vi "kill VSC debug port.vi"(8 "error in (no error)":errorcluster, 11 "vcd debug port (61558)":i32=61558) -> (0 "error out":errorcluster, 2 "pid killed":i32, 3 "vcd debug port out":i32)   [LabVIEW 2019]
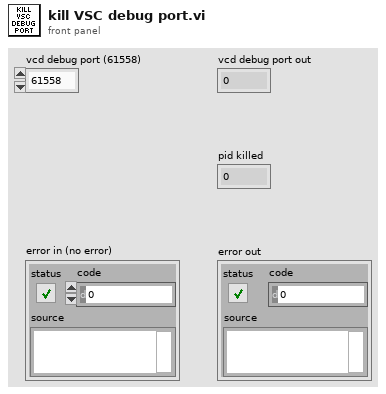
[diagram p1: front panel]
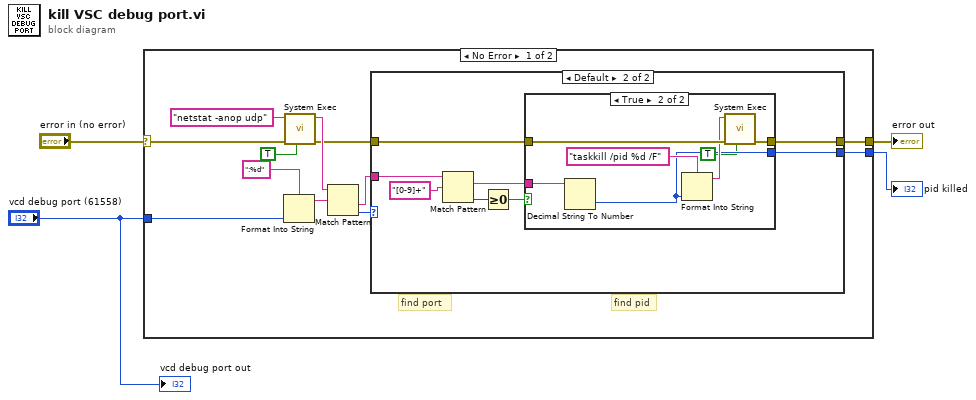
[diagram p0: block diagram]
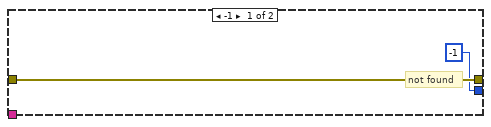
[diagram p2: hidden frame]
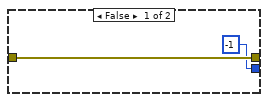
[diagram p3: hidden frame]
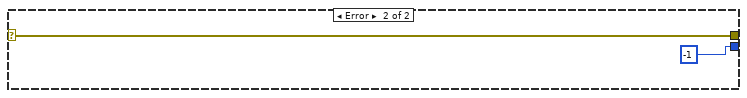
[diagram p4: hidden frame]
diagram:
  n1 = case shown="No Error" "error in (no error)" {
    selector: "error in (no error)" -> [w10 w37]
    tunnel: "vcd debug port (61558)" -> [w12 _]
    tunnel: [w7 w37] -> w3
    tunnel: [w6 -1] -> w2
    frame No Error {
      # "find pid"
      # "find port"
      n2 = Format Into String(format string=":%d", w12) -> (resulting string=w11:string)  [unwired: 2 in, 1 out]
      n3 = call <vilib>:"System Exec.vi"("run minimized? (F)"=TRUE, "error in (no error)"=w10, "command line"="netstat -anop udp") -> ("error out"=w8:errorcluster, "standard output"=w15:string)  [unwired: 5 in, 2 out]
      n4 = Match Pattern(string=w15, regular expression=w11) -> (after substring=w14:string, offset past match=w9:i32)  [unwired: 1 in, 2 out]
      n5 = case shown="Default" w9 {
        tunnel: w14 -> [_ w26]
        tunnel: w8 -> [w18 w24]
        tunnel: [w18 w23] -> w7
        tunnel: [-1 w19] -> w6
        frame -1 {
          # "not found"
        }
        frame Default {
          n6 = Match Pattern(string=w26, regular expression="[0-9]+" ("regular expression 2")) -> (match substring=w20:string, offset past match=w22:i32)  [unwired: 1 in, 2 out]
          n7 = Greater Or Equal To 0?(x=w22) -> (x >= 0?=w21:bool)
          n8 = case shown="True" w21 {
            tunnel: w24 -> [w28 w35]
            tunnel: [w28 w34] -> w23
            tunnel: w20 -> [_ w33]
            tunnel: [-1 w30] -> w19
            frame False {
            }
            frame True {
              n9 = Decimal String To Number(string=w33) -> (number=w30:i32)  [unwired: 2 in, 1 out]
              n10 = Format Into String(format string="taskkill /pid %d /F" ("command line 2"), w30) -> (resulting string=w31:string)  [unwired: 2 in, 1 out]
              n11 = call <vilib>:"System Exec.vi"("run minimized? (F)"=TRUE, "error in (no error)"=w35, "command line"=w31) -> ("error out"=w34:errorcluster)  [unwired: 5 in, 3 out]
            }
          }
        }
      }
    }
    frame Error {
    }
  }
  "error out" <- w3
  "pid killed" <- w2
  "vcd debug port out" <- "vcd debug port (61558)"
